vi "RtdeOutputDataReceivedCallbackVI.vi"(4 "Waveform Chart":refnum<vi>, 5 "Event Data":cluster{"sender":refnum<k24>, "e":refnum<k24>}, 6 "Control Ref":refnum<k24>, 7 "Event Common Data":T1) -> ()   [LabVIEW 2023]
uses:
  C:/Users/fg/Documents/UniversalRobots.vi/LabVIEW_2024/UnderAutomation.UniversalRobots/lib/UnderAutomation.UniversalRobots.dll
  LabVIEW_2024/UnderAutomation.UniversalRobots/lib/UnderAutomation.UniversalRobots.dll
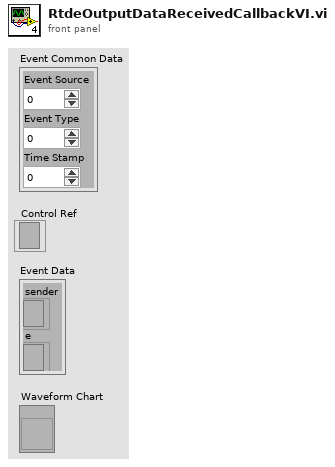
[diagram p1: front panel]
types:
  T1 = cluster{"Event Source":i32, "Event Type":u32, "Time Stamp":u32}
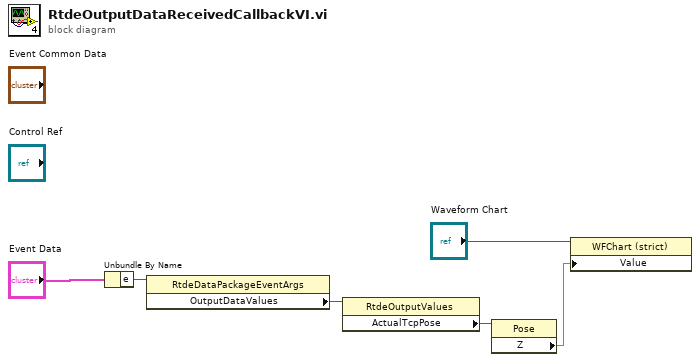
[diagram p0: block diagram]
diagram:
  n1 = Unbundle By Name("Event Data") -> ("e"=w5:refnum<k24>)
  n2 = property class="RtdeDataPackageEventArgs"(reference=w5) -> ("OutputDataValues"=w4:refnum<k24>)  [unwired: 1 in, 2 out]
  n3 = property class="RtdeOutputValues"(reference=w4) -> ("ActualTcpPose"=w3:refnum<k24>)  [unwired: 1 in, 2 out]
  n4 = property class="Pose"(reference=w3) -> ("Z"=w2:dbl)  [unwired: 1 in, 2 out]
  n5 = property class="WFChart (strict)"(reference="Waveform Chart", "Value"=w2) -> ()  [unwired: 1 in, 2 out]
